vi "Save VI.vi"(8 "error in (no error)":errorcluster, 10 "Ctl Properties":T1[](array[typedef]), 11 "VI Properties":T2) -> (0 "error out":errorcluster, 2 "Saved?":bool, 3 "VI Ref":refnum<vi>)   [LabVIEW 2023, in "VI Properties Editor.lvlib"]
doc: "Saves a VI based with <B>VI Properties</B> and <B>Ctl Properties</B>."
uses:
  VI Properties Editor.lvlib
  CTLs/VI Properties.ctl
  <vilib>/picture/picture.llb/imagedata.ctl
  CTLs/Control Properties.ctl
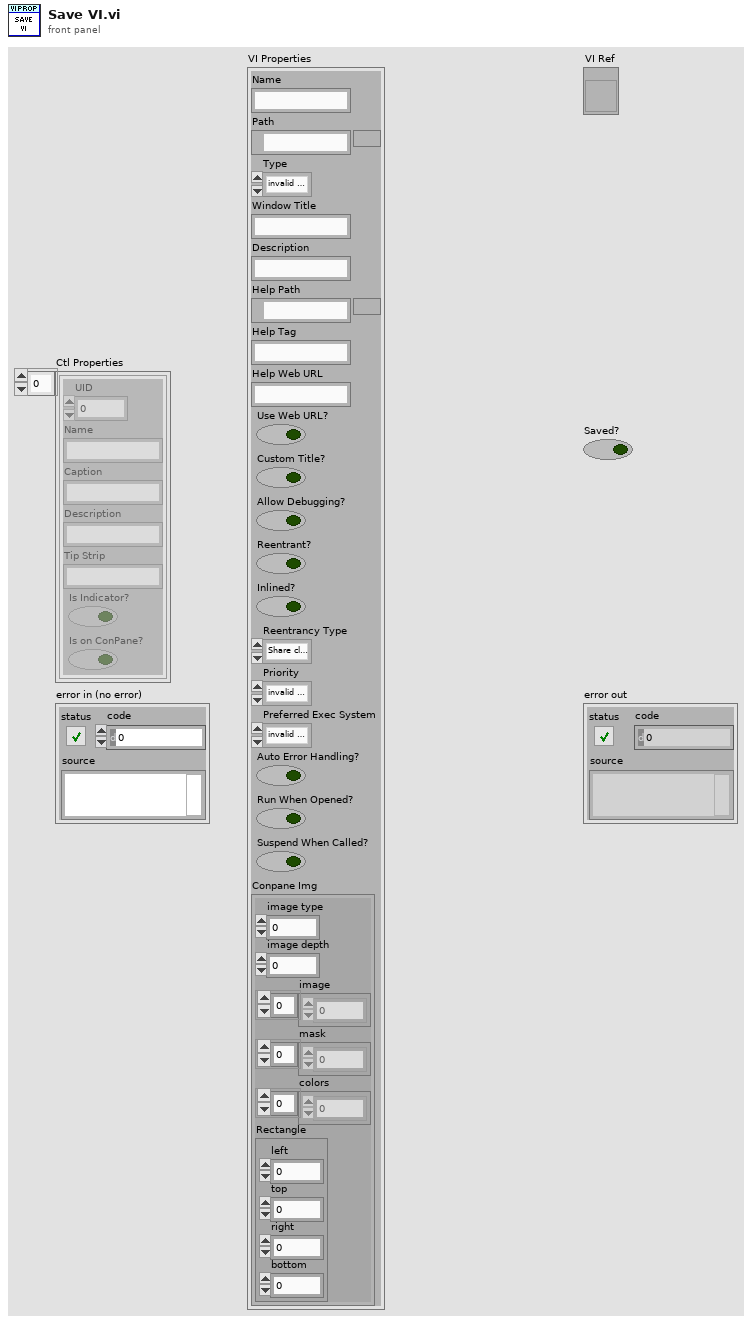
[diagram p1: front panel]
types:
  T1 = typedef "VI Properties Editor.lvlib/Control Properties.ctl" = cluster{"UID":i32, "Name":string, "Caption":string, "Description":string, "Tip Strip":string, "Is Indicator?":bool, "Is on ConPane?":bool}
  T2 = typedef "VI Properties Editor.lvlib/VI Properties.ctl" = cluster{"Name":string, "Path":path, "Type":enum32{"invalid VI type", "Standard VI", "Control VI", "Global VI", "Polymorphic VI", "Configuration VI", "SubSystem", "Facade VI", "Method VI", "Statechart Diagram VI"}, "Window Title":string, "Description":string, "Help Path":path, "Help Tag":string, "Help Web URL":string, "Use Web URL?":bool, "Custom Title?":bool, "Allow Debugging?":bool, "Reentrant?":bool, "Inlined?":bool, "Reentrancy Type":enum16{"Share clones between instances", "Preallocate clone for each instance"}, "Priority":enum32{"invalid priority", "background priority", "normal priority", "above normal priority", "high priority", "time critical priority", "subroutine"}, "Preferred Exec System":enum32{"invalid execution system", "user interface", "standard", "instrument i/o", "data acquisition", "other 1", "other 2", "same as caller"}, "Auto Error Handling?":bool, "Run When Opened?":bool, "Suspend When Called?":bool, "Conpane Img":T3}
  T3 = typedef "imagedata.ctl" = cluster{"image type":i32, "image depth":i32, "image":u8[], "mask":u8[], "colors":u32[], "Rectangle":cluster{"left":i16, "top":i16, "right":i16, "bottom":i16}}
  T4 = enum32{"invalid VI type", "Standard VI", "Control VI", "Global VI", "Polymorphic VI", "Configuration VI", "SubSystem", "Facade VI", "Method VI", "Statechart Diagram VI"}
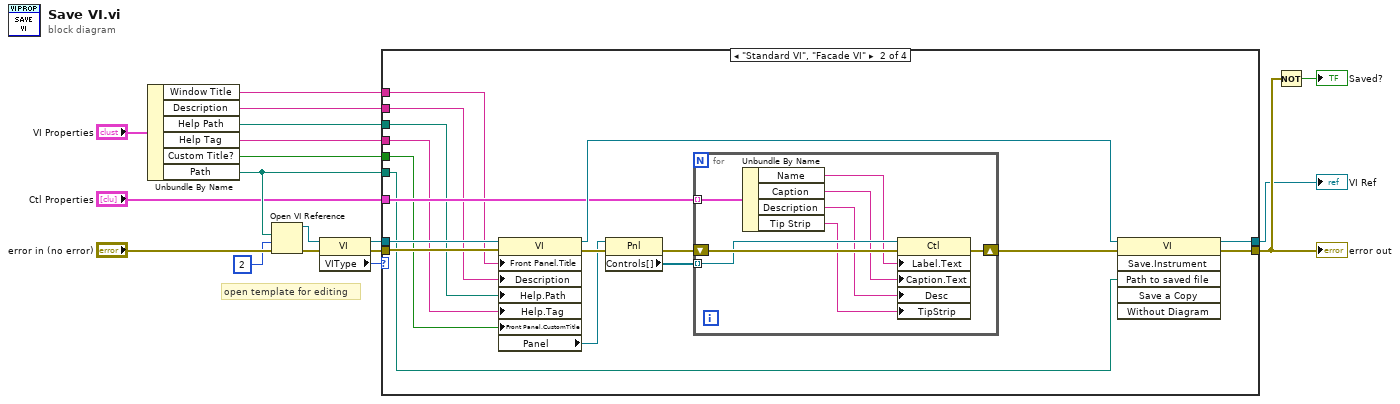
[diagram p0: block diagram]
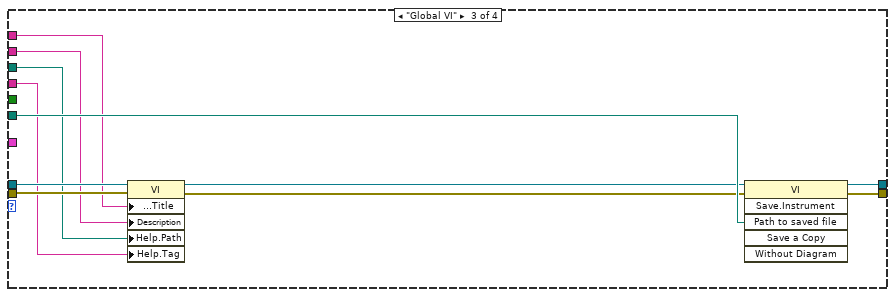
[diagram p3: hidden frame]
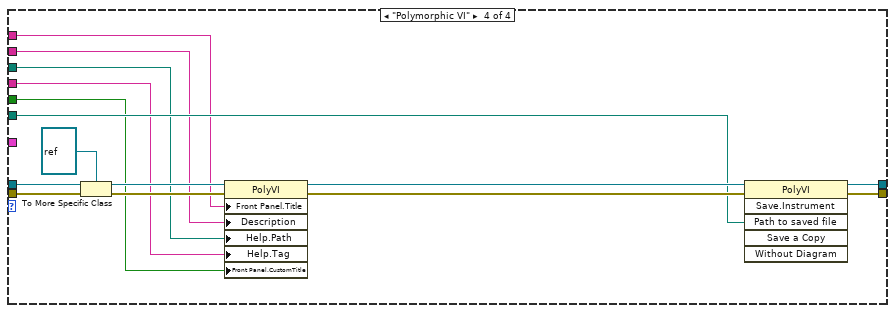
[diagram p4: hidden frame]
diagram:
  # "open template for editing"
  n1 = Unbundle By Name("VI Properties") -> ("Window Title"=w3:string, "Description"=w6:string, "Help Path"=w5:path, "Help Tag"=w7:string, "Custom Title?"=w2:bool, "Path"=w8:path)
  n2 = Open VI Reference(vi path=w8, options=2, error in (no error)="error in (no error)") -> (vi reference=w11:refnum<vi>, error out=w14:errorcluster)  [unwired: 3 in]
  n3 = property class="VI"(reference=w11, error in=w14) -> (reference out=w12:refnum<vi>, error out=w13:errorcluster, "VIType"=w15:T4)
  n4 = case shown="\"Standard VI\", \"Facade VI\"" w15 {
    tunnel: [w19 w37 w56 w71] -> w16
    tunnel: [w20 w36 w55 w70] -> w17
    tunnel: w12 -> [w19 w29 w51 w68]
    tunnel: w13 -> [w20 w28 w50 w67]
    tunnel: w6 -> [_ w26 w47 w58]
    tunnel: w7 -> [_ w24 w49 w59]
    tunnel: w5 -> [_ w23 w48 w60]
    tunnel: w8 -> [_ w22 w54 w62]
    tunnel: "Ctl Properties" -> [_ w27 _ _]
    tunnel: w3 -> [_ w25 w46 w57]
    tunnel: w2 -> [_ w21 _ w61]
    frame "invalid VI type", Default {
    }
    frame "Standard VI", "Facade VI" {
      n5 = property class="VI"(reference=w29, error in=w28, "Front Panel.Title"=w25, "Description"=w26, "Help.Path"=w23, "Help.Tag"=w24, "Front Panel.CustomTitle"=w21) -> (reference out=w32:refnum<vi>, error out=w35:errorcluster, "Panel"=w34:refnum<vi>)
      n6 = property class="Pnl"(reference=w34, error in=w35) -> (error out=w30:errorcluster, "Controls[]"=w31:refnum<vi>[])  [unwired: 1 out]
      n7 = for {
        tunnel: w31 -> [w43] mode=indexing
        shift-right: [w45] -> w33
        shift-left: w30 -> [w44]
        tunnel: w27 -> [w42] mode=indexing
        n8 = Unbundle By Name(w42) -> ("Name"=w41:string, "Caption"=w38:string, "Description"=w40:string, "Tip Strip"=w39:string)
        n9 = property class="Ctl"(reference=w43, error in=w44, "Label.Text"=w41, "Caption.Text"=w38, "Desc"=w40, "TipStrip"=w39) -> (error out=w45:errorcluster)  [unwired: 1 out]
      }
      n10 = invoke class="VI" method="Save.Instrument"(reference=w32, error in=w33, "Path to saved file"=w22) -> (reference out=w37:refnum<vi>, error out=w36:errorcluster)  [unwired: 3 in, 4 out]
    }
    frame "Global VI" {
      n11 = property class="VI"(reference=w51, error in=w50, "Front Panel.Title"=w46, "Description"=w47, "Help.Path"=w48, "Help.Tag"=w49) -> (reference out=w52:refnum<vi>, error out=w53:errorcluster)
      n12 = invoke class="VI" method="Save.Instrument"(reference=w52, error in=w53, "Path to saved file"=w54) -> (reference out=w56:refnum<vi>, error out=w55:errorcluster)  [unwired: 3 in, 4 out]
    }
    frame "Polymorphic VI" {
      n13 = To More Specific Class(target class=refnum<vi> refnum, reference=w68, error in=w67) -> (specific class reference=w66:refnum<vi>, error out=w65:errorcluster)
      n14 = property class="PolyVI"(reference=w66, error in=w65, "Front Panel.Title"=w57, "Description"=w58, "Help.Path"=w60, "Help.Tag"=w59, "Front Panel.CustomTitle"=w61) -> (reference out=w64:refnum<vi>, error out=w63:errorcluster)
      n15 = invoke class="PolyVI" method="Save.Instrument"(reference=w64, error in=w63, "Path to saved file"=w62) -> (reference out=w71:refnum<vi>, error out=w70:errorcluster)  [unwired: 3 in, 4 out]
    }
  }
  "error out" <- w17
  "VI Ref" <- w16
  n16 = Not(x=w17) -> (.not. x?=→"Saved?":bool)
